vi "NI-9203_SoftPanel.vi"(3 "NI-9203 in Slot:":string="1") -> ()   [LabVIEW 2016]
uses:
  HelperSubVIs/GlobalControlVariables.vi
panel:
  out "AI Values":dbl[](array[numeric])
  out "ExitModule":bool=TRUE
  out "AI 07":dbl
  out "AI 06":dbl
  out "AI 05":dbl
  out "AI 04":dbl
  out "AI 03":dbl
  out "AI 02":dbl
  out "AI 01":dbl
  out "AI 00":dbl
  in  "ExitButton":bool
  # "Analog Current Values (mA)"
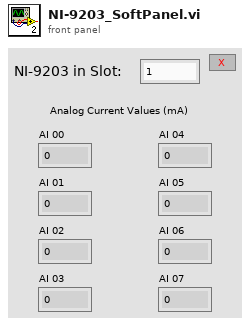
[diagram p1: front panel]
types:
  T1 = cluster{"AI Values[0]":dbl, "AI Values[1]":dbl, "AI Values[2]":dbl, "AI Values[3]":dbl, "AI Values[4]":dbl, "AI Values[5]":dbl, "AI Values[6]":dbl, "AI Values[7]":dbl}
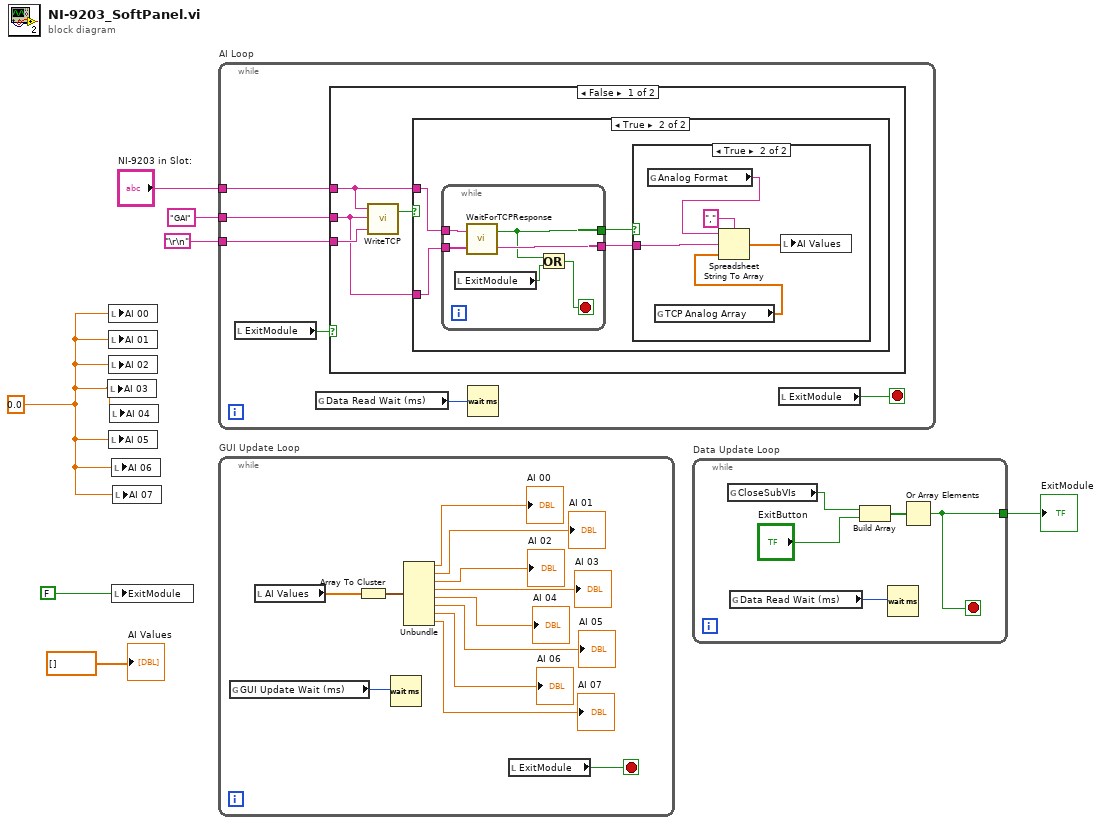
[diagram p0: block diagram]
diagram:
  w1 = 0.0
  n1 = local write "AI 03"(w1) -> ()
  n2 = local write "AI 00"(w1) -> ()
  n3 = local write "AI 01"(w1) -> ()
  n4 = local write "AI 02"(w1) -> ()
  n5 = local write "AI 05"(w1) -> ()
  n6 = local write "AI 04"(w1) -> ()
  n7 = local write "AI 06"(w1) -> ()
  n8 = local write "ExitModule"(FALSE) -> ()
  n9 = local write "AI 07"(w1) -> ()
  n10 = while "AI Loop" {
    tunnel: "NI-9203 in Slot:" -> [w12]
    tunnel: "\r\n" -> [w10]
    tunnel: "GAI" -> [w9]
    stop <- w13 stop-if-true
    n11 = local read "ExitModule"() -> (w8:bool)
    n12 = global read "GlobalControlVariables.vi" "Data Read Wait (ms)"() -> (w11:u32)
    n13 = case shown="False" w8 {
      tunnel: w12 -> [w16 _]
      tunnel: w10 -> [w15 _]
      tunnel: w9 -> [w14 _]
      frame False {
        n14 = call "WriteTCP.vi"("Data"=w15, "Action"=w14, "Module Slot"=w16) -> ("Sent"=w17:bool)  [unwired: 1 out]
        n15 = case shown="True" w17 {
          tunnel: w16 -> [_ w20]
          tunnel: w14 -> [_ w19]
          frame False {
          }
          frame True {
            n16 = while {
              tunnel: [w22] -> w21
              tunnel: w20 -> [w27]
              tunnel: w19 -> [w26]
              tunnel: [w25] -> w18
              stop <- w23 stop-if-true
              n17 = local read "ExitModule"() -> (w24:bool)
              n18 = call "WaitForTCPResponse.vi"("Action"=w26, "Module Slot"=w27) -> ("Received Data"=w25:string, "Ready"=w22:bool)
              n19 = Or(x=w22, y=w24) -> (x .or. y?=w23:bool)
            }
            n20 = case shown="True" w21 {
              tunnel: w18 -> [_ w32]
              frame False {
              }
              frame True {
                n21 = global read "GlobalControlVariables.vi" "Analog Format"() -> (w29:string)
                n22 = global read "GlobalControlVariables.vi" "TCP Analog Array"() -> (w30:dbl[])
                n23 = Spreadsheet String To Array(delimiter (Tab)=",", format string=w29, spreadsheet string=w32, array type (2D Dbl)=w30) -> (array=w28:dbl[])
                n24 = local write "AI Values"(w28) -> ()
              }
            }
          }
        }
      }
      frame True {
      }
    }
    n25 = Wait (ms)(milliseconds to wait=w11) -> ()  [unwired: 1 out]
    n26 = local read "ExitModule"() -> (w13:bool)
  }
  n27 = while "GUI Update Loop" {
    stop <- w33 stop-if-true
    n28 = global read "GlobalControlVariables.vi" "GUI Update Wait (ms)"() -> (w44:u32)
    n29 = local read "AI Values"() -> (w34:dbl[])
    n30 = Array To Cluster(array=w34) -> (cluster=w43:T1)
    n31 = Wait (ms)(milliseconds to wait=w44) -> ()  [unwired: 1 out]
    n32 = Unbundle(w43) -> ("AI Values[0]"=→"AI 00":dbl, "AI Values[1]"=→"AI 01":dbl, "AI Values[2]"=→"AI 02":dbl, "AI Values[3]"=→"AI 03":dbl, "AI Values[4]"=→"AI 04":dbl, "AI Values[5]"=→"AI 05":dbl, "AI Values[6]"=→"AI 06":dbl, "AI Values[7]"=→"AI 07":dbl)
    n33 = local read "ExitModule"() -> (w33:bool)
  }
  n34 = while "Data Update Loop" {
    tunnel: [w45] -> w7
    stop <- w45 stop-if-true
    n35 = global read "GlobalControlVariables.vi" "CloseSubVIs"() -> (w46:bool)
    n36 = global read "GlobalControlVariables.vi" "Data Read Wait (ms)"() -> (w49:u32)
    n37 = Build Array(w46, "ExitButton") -> (w48:bool[])
    n38 = Wait (ms)(milliseconds to wait=w49) -> ()  [unwired: 1 out]
    n39 = Or Array Elements(Boolean array=w48) -> (logical OR=w45:bool)
  }
  "ExitModule" <- w7
  "AI Values" <- dbl[] []
